vi "AutoScan.vi"(9 "menu reference":refnum<k9>, 10 "Information":refnum<vi>, 11 "Port 2":refnum<vi>) -> (0 "Process":T1, 2 "Information":refnum<vi>, 3 "reference out":refnum<vi>)   [LabVIEW 2013]
uses:
  Control/SystemProcess.ctl
  Control/Buffer.vi
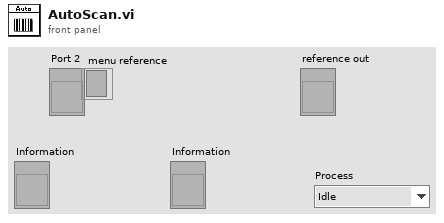
[diagram p1: front panel]
types:
  T1 = typedef "SystemProcess.ctl" = enum16{"Idle", "SystemInit", "SpecialEvent", "Barcode(SN)", "TestInitialize", "Test", "Stop", "SaveTestData", "Exit"}
  T2 = typedef "Port.ctl" = cluster{"Multimeter":refnum<visa-resource-name>, "ACsource ":refnum<visa-resource-name>, "GEA":refnum<visa-resource-name>, "LEDanalizer":refnum<visa-resource-name>, "AutoScan":refnum<visa-resource-name>, "lines":tag, "MabeCOM":refnum<visa-resource-name>}
  T3 = typedef "StatusInformation.ctl" = cluster{"FileName:":string, "Barcode(S/N):":string, "TestStep:":string, "TestTime:":string, "Station:":string, "Model:":string, "Line:":string, "Status:":string, "Series:":string, "Reserve:":string}
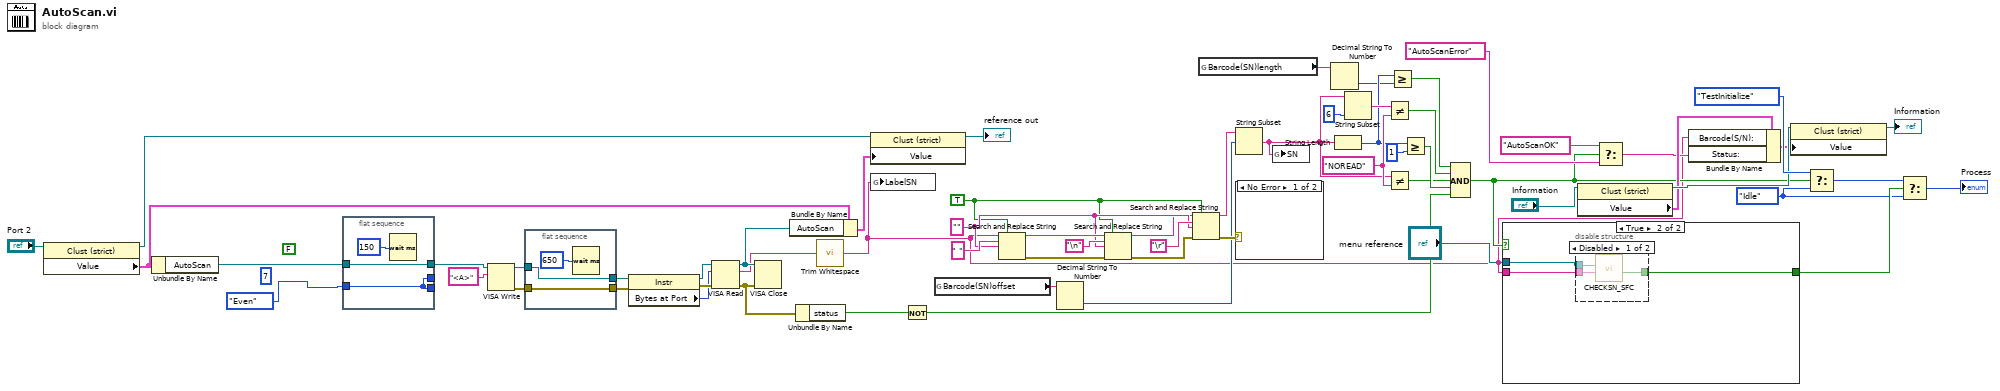
[diagram p0: block diagram]
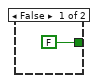
[diagram p2: hidden frame]
diagram:
  w20 = "NOREAD" ("y")
  w39 = "" ("search string")
  w36 = TRUE ("replace all? (F)")
  w7 = SystemProcess."Idle" ("f")
  (unwired) FALSE ("Enable Termination\nChar (T)")
  (unwired) u16 7 ("data bits (8)")
  n1 = property class="Clust (strict)"(reference="Port 2") -> (reference out=w48:refnum<vi>, "Value"=w47:T2)  [unwired: 1 in, 1 out]
  n2 = Unbundle By Name(w47) -> ("AutoScan"=w1:refnum<visa-resource-name>)
  n3 = flat-sequence {
    tunnel: [w65] -> w54
    tunnel: w1 -> [w65]
    tunnel: [w63] -> _
    tunnel: [w63] -> _
    tunnel: enum16{"None", "Odd", "Even", "Mark", "Space"}."Even" ("parity (0:none)") -> [w63]
    frame #0 {
      n4 = Wait (ms)(milliseconds to wait=u32 150) -> ()  [unwired: 1 out]
    }
  }
  n5 = VISA Write(VISA resource name=w54, write buffer="<A>") -> (VISA resource name out=w61:refnum<visa-resource-name>, error out=w60:errorcluster)  [unwired: 1 in, 1 out]
  n6 = flat-sequence {
    tunnel: [w68] -> w59
    tunnel: w61 -> [w68]
    tunnel: w60 -> [w67]
    tunnel: [w67] -> w58
    frame #0 {
      n7 = Wait (ms)(milliseconds to wait=u32 650) -> ()  [unwired: 1 out]
    }
  }
  n8 = property class="Instr"(reference=w59, error in=w58) -> (reference out=w56:refnum<visa-resource-name>, error out=w57:errorcluster, "Bytes at Port"=w55:u32)
  n9 = VISA Read(VISA resource name=w56, byte count=w55, error in (no error)=w57) -> (VISA resource name out=w18:refnum<visa-resource-name>, read buffer=w3:string, error out=w17:errorcluster)  [unwired: 1 out]
  n10 = VISA Close(VISA resource name=w18, error in (no error)=w17) -> ()  [unwired: 1 out]
  n11 = Bundle By Name(cluster=w47, "AutoScan"=w18) -> (w46:T2)
  n12 = Unbundle By Name(w17) -> ("status"=w51:bool)
  n13 = call <vilib>:"Trim Whitespace.vi"("string"=w3) -> ("trimmed string"=w4:string)  [unwired: 1 in]
  n14 = property class="Clust (strict)"(reference=w48, "Value"=w46) -> (reference out=→"reference out":refnum<vi>)  [unwired: 1 in, 1 out]
  n15 = global write "Buffer.vi" "LabelSN"(w4) -> ()
  n16 = Not(x=w51) -> (.not. x?=w50:bool)
  n17 = global read "Buffer.vi" "Barcode(SN)offset"() -> (w26:string)
  n18 = Search and Replace String(replace all?=w36, input string=w4, search string=" ", replace string=w39) -> (result string=w44:string, error out=w43:errorcluster)  [unwired: 4 in, 2 out]
  n19 = Decimal String To Number(string=w26) -> (number=w25:i32)  [unwired: 2 in, 1 out]
  n20 = Search and Replace String(replace all?=w36, input string=w44, search string="\n", replace string=w39, error in=w43) -> (result string=w37:string, error out=w40:errorcluster)  [unwired: 3 in, 2 out]
  n21 = Search and Replace String(replace all?=w36, input string=w37, search string="\r", replace string=w39, error in=w40) -> (result string=w23:string, error out=w38:errorcluster)  [unwired: 3 in, 2 out]
  n22 = global read "Buffer.vi" "Barcode(SN)length"() -> (w24:string)
  n23 = String Subset(string=w23, offset (0)=w25) -> (substring=w16:string)  [unwired: 1 in]
  n24 = case shown="No Error" w38 {
    frame No Error {
    }
    frame Error {
    }
  }
  n25 = global write "Buffer.vi" "SN"(w16) -> ()
  n26 = Decimal String To Number(string=w24) -> (number=w14:i32)  [unwired: 2 in, 1 out]
  n27 = String Length(string=w16) -> (length=w15:i32)
  n28 = String Subset(string=w16, length (rest)=6 ("length (rest)")) -> (substring=w21:string)  [unwired: 1 in]
  n29 = Not Equal?(x=w21, y=w20) -> (x != y?=w19:bool)
  n30 = Not Equal?(x=w16, y=w20) -> (x != y?=w27:bool)
  n31 = Greater Or Equal?(x=w15, y=w14) -> (x >= y?=w13:bool)
  n32 = Greater Or Equal?(x=w15, y=1) -> (x >= y?=w49:bool)
  n33 = Compound Arithmetic op=AND(w13, w19, w27, w49, w50) -> (w5:bool)
  n34 = case shown="True" w5 {
    tunnel: [FALSE ("SNCheck") w72] -> w8
    tunnel: w4 -> [_ w71]
    tunnel: "menu reference" -> [_ w70]
    frame False {
    }
    frame True {
      n35 = disable-structure shown="Disabled" {
        disable-tunnel: [w75 _] -> w72
        disable-tunnel: w71 -> [w74 _]
        disable-tunnel: w70 -> [w73 _]
        frame Disabled {
          n36 = call "CHECKSN_SFC.vi"("SN"=w74, "menu reference"=w73) -> ("SNCheck"=w75:bool)  [unwired: 8 in, 1 out]
        }
        frame Enabled {
        }
      }
    }
  }
  n37 = property class="Clust (strict)"(reference="Information") -> (reference out=w33:refnum<vi>, "Value"=w29:T3)  [unwired: 1 in, 1 out]
  n38 = Select(t="AutoScanOK", s=w5, f="AutoScanError") -> (s? t:f=w28:string)
  n39 = Bundle By Name(cluster=w29, "Barcode(S/N):"=w4, "Status:"=w28) -> (w30:T3)
  n40 = property class="Clust (strict)"(reference=w33, "Value"=w30) -> (reference out=→"Information":refnum<vi>)  [unwired: 1 in, 1 out]
  n41 = Select(t=SystemProcess."TestInitialize" ("MainProcess"), s=w5, f=w7) -> (s? t:f=w10:T1)
  n42 = Select(t=w10, s=w8, f=w7) -> (s? t:f=→"Process":T1)
